vi "Select Printer.vi"(8 "error in (no error)":errorcluster) -> (0 "error out":errorcluster, 3 "Canceled?":bool=TRUE)   [LabVIEW 2011]
panel:
  in  "Printers":i32(listbox)=-1
  in  "Cancel":bool
  in  "OK":bool
  # "Please select a printer to use:"
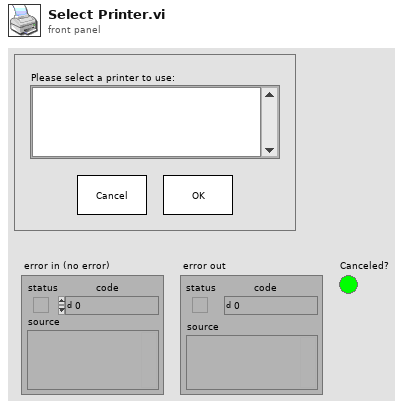
[diagram p1: front panel]
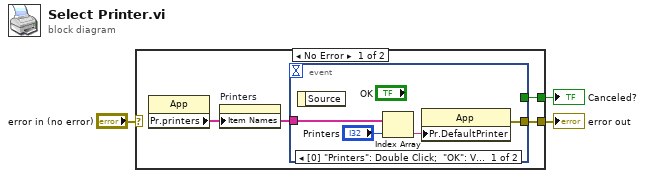
[diagram p0: block diagram]
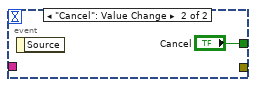
[diagram p2: hidden frame]
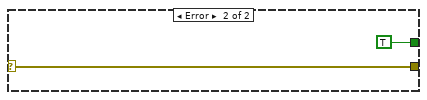
[diagram p3: hidden frame]
diagram:
  n1 = case shown="No Error" "error in (no error)" {
    selector: "error in (no error)" -> [_ w13]
    tunnel: [w6 w13] -> w3
    tunnel: [w5 TRUE ("Cancel")] -> w1
    frame No Error {
      n2 = property class="App"() -> ("Pr.printers"=w4:string[])  [unwired: 2 in, 2 out]
      n3 = property on="Printers" class="LstBox (strict)"("Item Names"=w4) -> ()  [unwired: 2 in, 2 out]
      n4 = event shown="[0] \"Printers\": Double Click;  \"OK\": Value Change" {
        selector: _ -> [_ _]
        dyn-events: _ -> [_ _]
        timeout: _ -> [_ _]
        tunnel: w4 -> [w8 _]
        tunnel: [_ "Cancel"] -> w5
        tunnel: [w7 _] -> w6
        event "Printers": Double Click; "OK": Value Change {
          n5 = event-data() -> ()  [unwired: 2 out]
          n6 = Index Array(array=w8, index="Printers") -> (element=w10:string)
          n7 = property class="App"("Pr.DefaultPrinter"=w10) -> (error out=w7:errorcluster)  [unwired: 2 in, 1 out]
        }
        event "Cancel": Value Change {
          n8 = event-data() -> ()  [unwired: 2 out]
        }
      }
    }
    frame Error {
    }
  }
  "error out" <- w3
  "Canceled?" <- w1
